vi "Activity_4.vi"() -> ()   [LabVIEW 2015]
panel:
  in  "stop":bool
  in  "Ring":u16(ring)=4 items=["Totodile", "Sceptile", "Rayquaza", "Swampert", "Houndoom", "Garchomp"]
  # "Menu Ring con Imágenes y Texto"
  # "Fecha de Entrega: 9/2/2019"
  # "Serrano Bermúdez Luis Esteban"
  # "Descripción:"
  # "Este programa crea un menu de imágenes\ny texto"
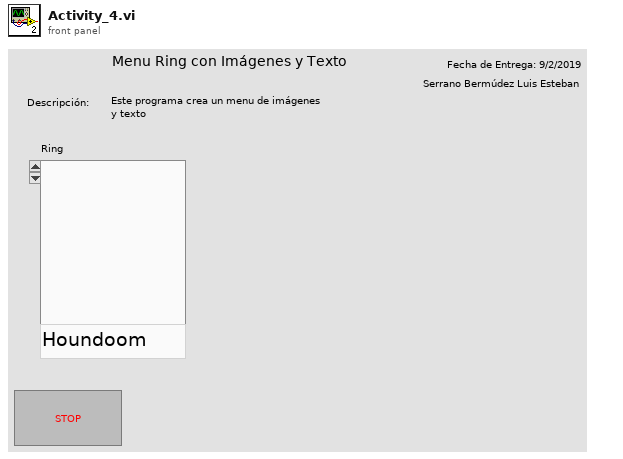
[diagram p1: front panel]
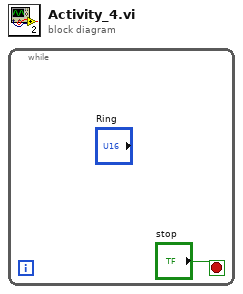
[diagram p0: block diagram]
diagram:
  n1 = while {
    stop <- "stop" stop-if-true
  }
